vi "Configure Scale.vi"(5 "Scaling Function (0: dB)":i32(ring) items=["dB", "dBM", "PCT", "Scale"], 6 "Enable Scaling (F: Disable)":bool, 7 "Auto Reference (T: Enable)":bool=TRUE, 8 "error in (no error)":errorcluster, 9 "Reference Resistance (600 ohms)":i32(ring)=600 items=["2"=2, "4"=4, "8"=8, "16"=16, "50"=50, "75"=75, "93"=93, "110"=110, "124"=124, "125"=125, "135"=135, "150"=150, "250"=250, "300"=300, "500"=500, "600"=600, "800"=800, "900"=900, "1000"=1000, "1200"=1200, "8000"=8000], 10 "Relative Value (0 dBm)":dbl, 11 "VISA resource name":refnum<visa-resource-name>) -> (0 "error out":errorcluster, 3 "VISA resource name out":refnum<visa-resource-name>)   [LabVIEW 2020, in "Agilent 3446X Series.lvlib"]
doc: "Configures scale settings.\n\n<b>Note(s) : </b>\nThis VI applies only to ACV and DCV measurement functions."
uses:
  <instrlib>/Agilent 3446X Series/Agilent 3446X Series.lvlib
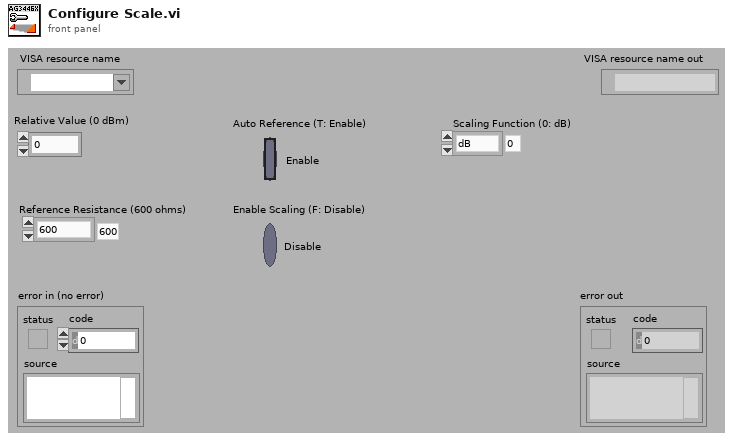
[diagram p1: front panel]
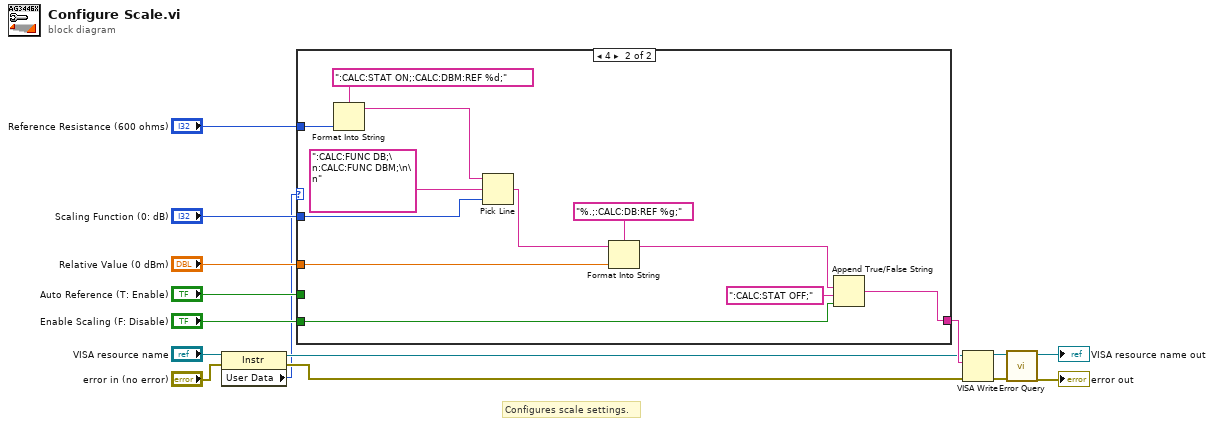
[diagram p0: block diagram]
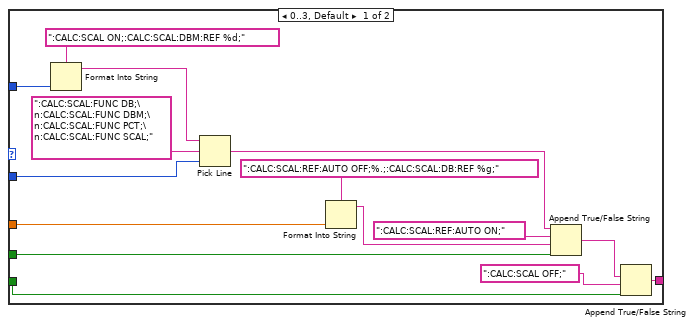
[diagram p2: hidden frame]
diagram:
  # "Configures scale settings."
  n1 = property class="Instr"(reference="VISA resource name", error in="error in (no error)") -> (reference out=w3:refnum<visa-resource-name>, error out=w2:errorcluster, "User Data"=w1:u32)
  n2 = case shown="4" w1 {
    tunnel: "Relative Value (0 dBm)" -> [w29 w35]
    tunnel: "Reference Resistance (600 ohms)" -> [w27 w37]
    tunnel: "Scaling Function (0: dB)" -> [w25 w36]
    tunnel: "Auto Reference (T: Enable)" -> [w24 _]
    tunnel: "Enable Scaling (F: Disable)" -> [w22 w34]
    tunnel: [w21 w33] -> w10
    frame 0..3, Default {
      n3 = Format Into String(format string=":CALC:SCAL ON;:CALC:SCAL:DBM:REF %d;", w27) -> (resulting string=w19:string)  [unwired: 2 in, 1 out]
      n4 = Pick Line(string ("")=w19, multi-line string=":CALC:SCAL:FUNC DB;\n:CALC:SCAL:FUNC DBM;\n:CALC:SCAL:FUNC PCT;\n:CALC:SCAL:FUNC SCAL;", line index=w25) -> (output string=w17:string)
      n5 = Format Into String(format string=":CALC:SCAL:REF:AUTO OFF;%.;:CALC:SCAL:DB:REF %g;", w29) -> (resulting string=w20:string)  [unwired: 2 in, 1 out]
      n6 = Append True/False String(1:w24, 2:w20, 3:":CALC:SCAL:REF:AUTO ON;", 4:w17) -> (0:w16:string)
      n7 = Append True/False String(1:w22, 2:":CALC:SCAL OFF;", 3:w16) -> (0:w21:string)  [unwired: 1 out]
    }
    frame 4 {
      n8 = Format Into String(format string=":CALC:STAT ON;:CALC:DBM:REF %d;", w37) -> (resulting string=w39:string)  [unwired: 2 in, 1 out]
      n9 = Pick Line(string ("")=w39, multi-line string=":CALC:FUNC DB;\n:CALC:FUNC DBM;\n\n", line index=w36) -> (output string=w32:string)
      n10 = Format Into String(format string="%.;:CALC:DB:REF %g;", initial string=w32, w35) -> (resulting string=w31:string)  [unwired: 1 in, 1 out]
      n11 = Append True/False String(1:w34, 2:":CALC:STAT OFF;", 3:w31) -> (0:w33:string)  [unwired: 1 out]
    }
  }
  n12 = VISA Write(VISA resource name=w3, write buffer=w10, error in (no error)=w2) -> (VISA resource name out=w9:refnum<visa-resource-name>, error out=w8:errorcluster)  [unwired: 1 out]
  n13 = call <instrlib>:"Error Query.vi"("error in (no error)"=w8, "VISA resource name"=w9) -> ("error out"=→"error out":errorcluster, "VISA resource name out"=→"VISA resource name out":refnum<visa-resource-name>)  [unwired: 8 out]
